vi "SP Format Ch Plot Label.vi"(6 "Channel":i8=1 min=1 max=99 step=1, 8 "error in (no error)":errorcluster, 9 "CH Controls":T1={"Trace On"=TRUE, "Measure"=0, "Format"=0, "Autoscale"=TRUE, "Reference"=0.0, "\nRefUnit"="dB/Div", "Position"=5.0, "Scale"=10.0, "ScaleUnit"="dB/Div", "LimitOn"=TRUE, "LimitFill"=FALSE, "Display Data"=0, "Show Markers"=TRUE, "SXX"=""} {"Reference" format="%#.2g"; "Display Data" items=["Data", "Memory", "Data/Memory"]; "Format" items=["Log Mag", "Phase", "Expanded Phase", "Delay", "Smith", "Polar", "Lin Mag", "SWR", "Loss", "Real", "Imaginary"]; "Scale" min=0.001 step=1.0 format="%#.2g"; "Position" min=0.0 max=10.0}, 11 "Plot Reference":refnum<vi>) -> (0 "error out":errorcluster, 1 "dup CH Controls":T1={"Trace On"=TRUE, "Measure"=0, "Format"=0, "Autoscale"=TRUE, "Reference"=0.0, "\nRefUnit"="dB/Div", "Position"=5.0, "Scale"=10.0, "ScaleUnit"="dB/Div", "LimitOn"=TRUE, "LimitFill"=FALSE, "Display Data"=0, "Show Markers"=TRUE, "SXX"=""} {"Reference" format="%#.2g"; "Display Data" items=["Data", "Memory", "Data/Memory"]; "Format" items=["Log Mag", "Phase", "Expanded Phase", "Delay", "Smith", "Polar", "Lin Mag", "SWR", "Loss", "Real", "Imaginary"]; "Scale" min=0.001 step=1.0 format="%#.2g"; "Position" min=0.0 max=10.0}, 3 "Plot Reference":refnum<vi>)   [LabVIEW 2011]
uses:
  TypeDefs/SP Display Trace Controls.ctl
  TypeDefs/SP Display Format.ctl
  TypeDefs/SP Display Data.ctl
  TypeDefs/SP Plot Cluster Object.ctl
panel:
  # "Div"
  # "Div"
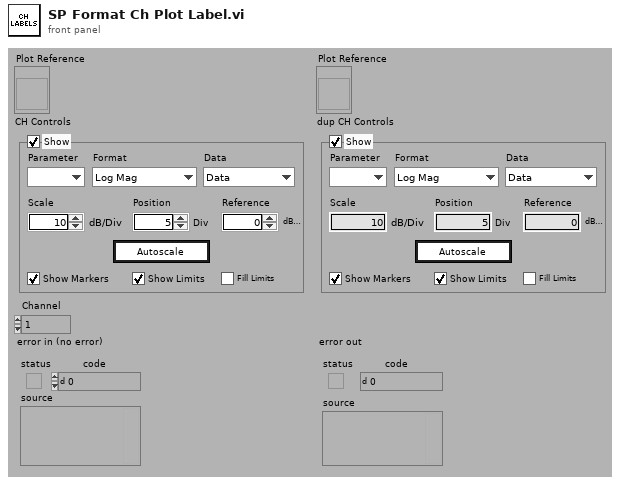
[diagram p1: front panel]
types:
  T1 = typedef "SP Display Trace Controls.ctl" = cluster{"Trace On":bool, "Measure":i32, "Format":T2, "Autoscale":bool, "Reference":dbl, "\nRefUnit":string, "Position":dbl, "Scale":dbl, "ScaleUnit":string, "LimitOn":bool, "LimitFill":bool, "Display Data":T3, "Show Markers":bool, "SXX":string}
  T2 = typedef "SP Display Format.ctl" = i32
  T3 = typedef "SP Display Data.ctl" = u16
  T4 = typedef "SP Plot Cluster Object.ctl" = enum16{"Plot", "CH Reference", "CH Label", "Start Label", "Stop Label", "Units Label", "Selected?", "CH Markers"}
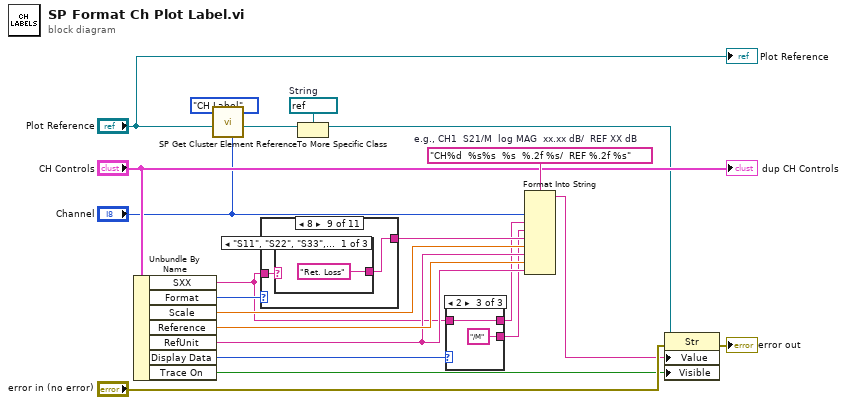
[diagram p0: block diagram]
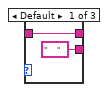
[diagram p2: hidden frame]
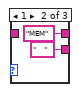
[diagram p3: hidden frame]
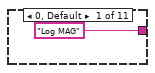
[diagram p4: hidden frame]
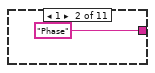
[diagram p5: hidden frame]
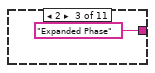
[diagram p6: hidden frame]
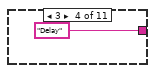
[diagram p7: hidden frame]
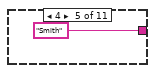
[diagram p8: hidden frame]
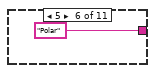
[diagram p9: hidden frame]
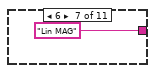
[diagram p10: hidden frame]
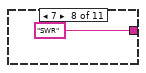
[diagram p11: hidden frame]
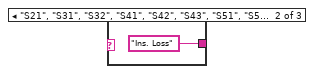
[diagram p12: hidden frame]
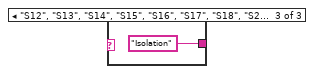
[diagram p13: hidden frame]
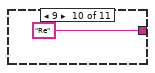
[diagram p14: hidden frame]
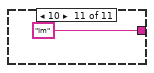
[diagram p15: hidden frame]
diagram:
  w7 = refnum<vi> refnum  # String
  w19 = "CH%d  %s%s  %s  %.2f %s/  REF %.2f %s"  # e.g., CH1  S21/M  log MAG  xx.xx dB/  REF XX dB
  n1 = Unbundle By Name("CH Controls") -> ("SXX"=w1:string, "Format"=w17:T2, "Scale"=w12:dbl, "Reference"=w14:dbl, "RefUnit"=w13:string, "Display Data"=w10:T3, "Trace On"=w15:bool)
  n2 = call "SP Get Cluster Element Reference.vi"("Channel"="Channel", "Element"=SP_Plot_Cluster_Object."CH Label", "Plot Reference"="Plot Reference") -> ("Element Reference"=w6:refnum<vi>)  [unwired: 6 out]
  n3 = case shown="8" w17 {
    tunnel: ["Log MAG" "Phase" "Expanded Phase" "Delay" "Smith" "Polar" "Lin MAG" "SWR" w30 "Re" "Im"] -> w11
    tunnel: w1 -> [_ _ _ _ _ _ _ _ w31 _ _]
    frame 0, Default {
    }
    frame 1 {
    }
    frame 2 {
    }
    frame 3 {
    }
    frame 4 {
    }
    frame 5 {
    }
    frame 6 {
    }
    frame 7 {
    }
    frame 8 {
      n4 = case shown="\"S11\", \"S22\", \"S33\", \"S44\", \"S55\", \"S66\", \"S77\", \"S88\", Default" w31 {
        tunnel: ["Ret. Loss" "Ins. Loss" "Isolation"] -> w30
        frame "S11", "S22", "S33", "S44", "S55", "S66", "S77", "S88", Default {
        }
        frame "S21", "S31", "S32", "S41", "S42", "S43", "S51", "S52", "S53", "S54", "S61", "S62", "S63", "S64", "S65", "S71", "S72", "S73", "S74", "S75", "S76", "S81", "S82", "S83", "S84", "S85", "S86", "S87" {
        }
        frame "S12", "S13", "S14", "S15", "S16", "S17", "S18", "S23", "S24", "S25", "S26", "S27", "S28", "S34", "S35", "S36", "S37", "S38", "S45", "S46", "S47", "S48", "S56", "S57", "S58", "S67", "S68", "S78" {
        }
      }
    }
    frame 9 {
    }
    frame 10 {
    }
  }
  n5 = To More Specific Class(target class=w7, reference=w6) -> (specific class reference=w5:refnum<vi>)  [unwired: 1 in, 1 out]
  n6 = case shown="2" w10 {
    tunnel: w1 -> [w38 _ w41]
    tunnel: [w38 "MEM" w41] -> w9
    tunnel: ["     " "    " "/M"] -> w8
    frame Default {
    }
    frame 1 {
    }
    frame 2 {
    }
  }
  n7 = Format Into String(format string=w19, "Channel", w9, w8, w11, w12, w13, w14, w13) -> (resulting string=w18:string)  [unwired: 2 in, 1 out]
  n8 = property class="Str"(reference=w5, error in="error in (no error)", "Value"=w18, "Visible"=w15) -> (error out=→"error out":errorcluster)  [unwired: 1 out]
  "dup CH Controls" <- "CH Controls"
  "Plot Reference" <- "Plot Reference"
